vi "mini.vi"(8 "error in (no error)":errorcluster, 9 "stop":bool, 10 "queue out 2":refnum<queue>, 11 "connection ID 2":refnum<k5>) -> (0 "error out 3":errorcluster, 2 "queue out":refnum<queue>, 3 "connection ID":refnum<k5>)   [LabVIEW 2017]
uses:
  gloabal.vi
panel:
  in  "address":string="192.168.10.23"
  in  "timeout (ms)":i32=10000
  in  "bytes to read":i32=1280
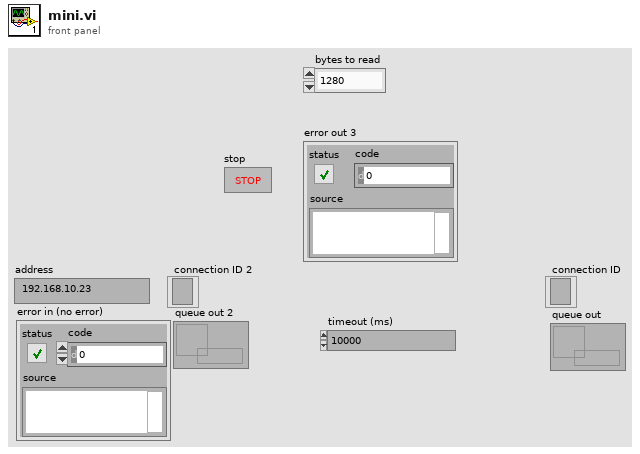
[diagram p1: front panel]
types:
  T1 = enum16{"Standard", "Buffered", "CRLF", "Immediate"}
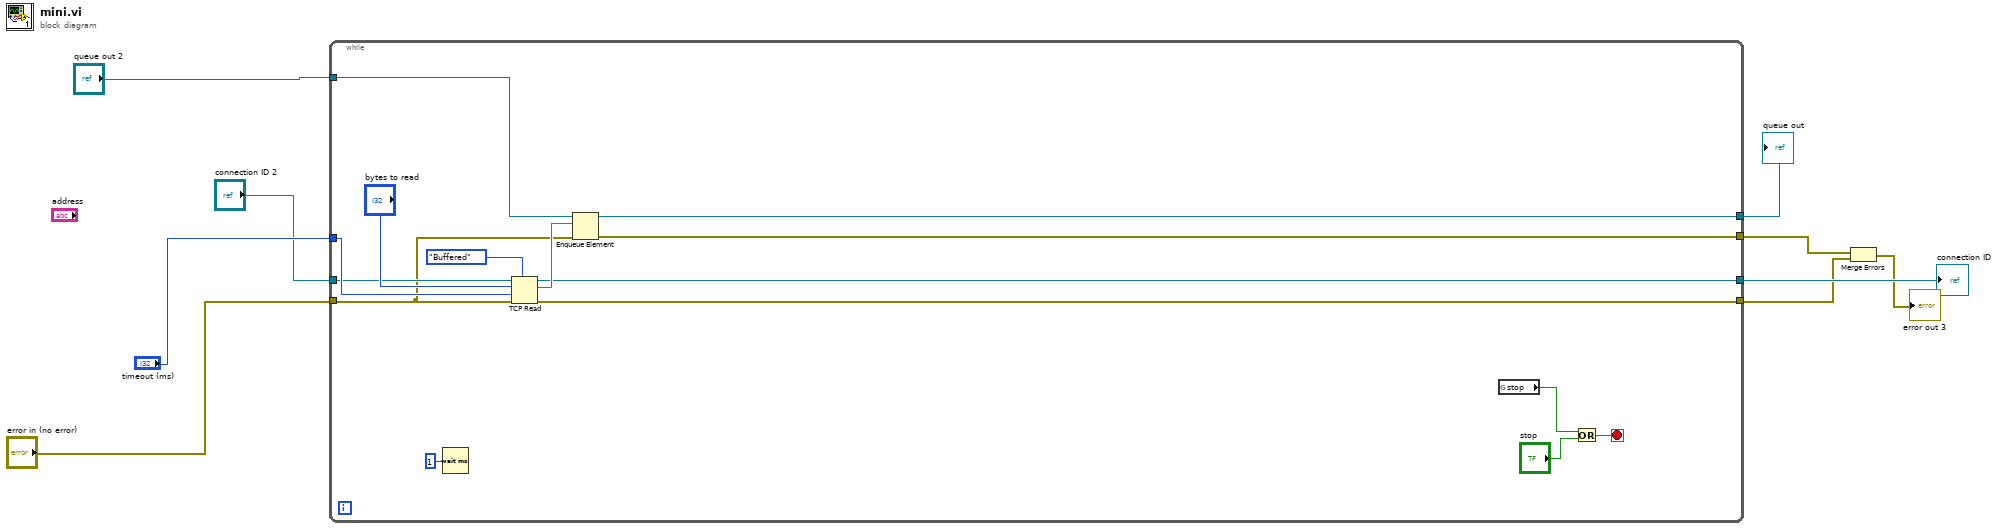
[diagram p0: block diagram]
diagram:
  n1 = while {
    tunnel: "queue out 2" -> [w24]
    tunnel: "error in (no error)" -> [w13]
    tunnel: "timeout (ms)" -> [w22]
    tunnel: "connection ID 2" -> [w21]
    tunnel: [w19] -> w9
    tunnel: [w18] -> w6
    tunnel: [w16] -> w8
    tunnel: [w15] -> w4
    stop <- w11 stop-if-true
    n2 = Wait (ms)(milliseconds to wait=u32 1) -> ()  [unwired: 1 out]
    n3 = TCP Read(connection ID=w21, bytes to read="bytes to read", error in (no error)=w13, 7:T1."Buffered" ("mode (standard)"), 9:w22) -> (connection ID out=w19:refnum<k5>, data out=w20:string, error out=w18:errorcluster)
    n4 = Enqueue Element(queue=w24, element=w20, error in (no error)=w13) -> (queue out=w16:refnum<queue>, error out=w15:errorcluster)  [unwired: 1 in, 1 out]
    n5 = global read "gloabal.vi" "stop"() -> (w10:bool)
    n6 = Or(x=w10, y="stop") -> (x .or. y?=w11:bool)
  }
  "connection ID" <- w9
  "queue out" <- w8
  n7 = Merge Errors(w4, w6) -> (→"error out 3":errorcluster)
